vi "CODcr测量数据区.vi"(11 "数组":u16[](array[numeric]) format="%04xH") -> (3 "测量数据区":T1 {"单位" items=["ug/L", "mg/L", "ppm", "mg/m3", "cm", "ppb", "ug/m3", "%", "nmol/mol", "umol/mol", "MPN/L", "MPN/100ml", "ng/m3", "NTU", "无量纲", "ms/cm", "us/cm", "℃", "mV", "万个/L"]})   [LabVIEW 2016, in "CODCr库.lvlib"]
panel:
  # "共占用95 WORD"
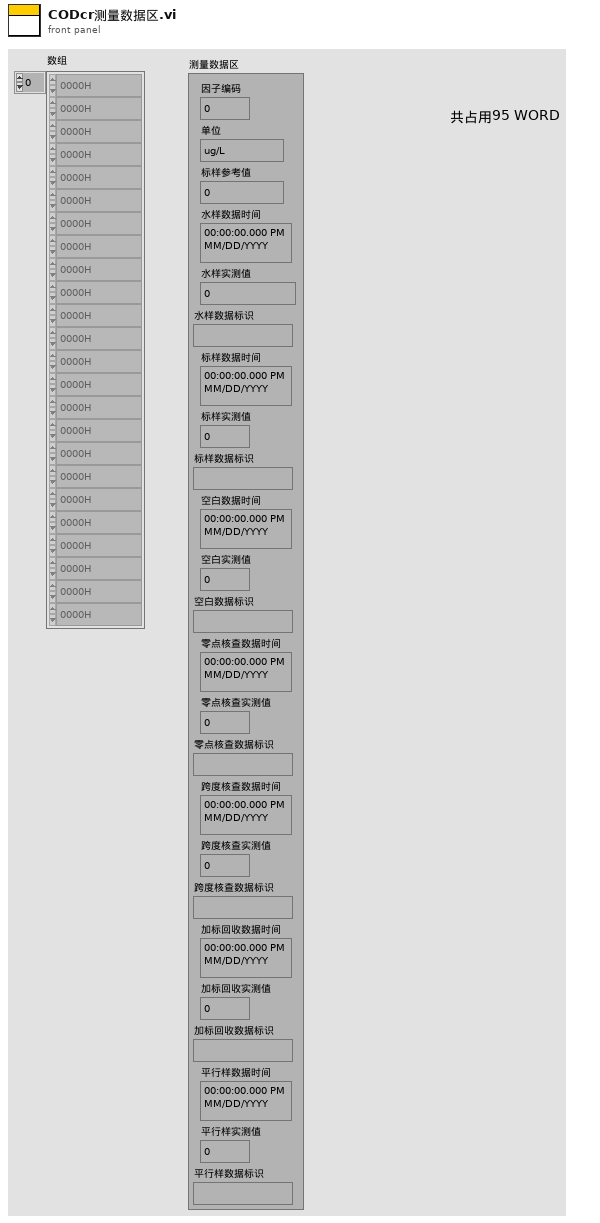
[diagram p1: front panel]
types:
  T1 = cluster{"因子编码":u32, "单位":u16, "标样参考值":sgl, "水样数据时间":timestamp, "水样实测值":sgl, "水样数据标识":string, "标样数据时间":timestamp, "标样实测值":sgl, "标样数据标识":string, "空白数据时间":timestamp, "空白实测值":sgl, "空白数据标识":string, "零点核查数据时间":timestamp, "零点核查实测值":sgl, "零点核查数据标识":string, "跨度核查数据时间":timestamp, "跨度核查实测值":sgl, "跨度核查数据标识":string, "加标回收数据时间":timestamp, "加标回收实测值":sgl, "加标回收数据标识":string, "平行样数据时间":timestamp, "平行样实测值":sgl, "平行样数据标识":string}
  T2 = cluster{"DWORD":i32, "WORD":u16, "FLOAT":sgl, "time stamp":timestamp, "数值":sgl, "string":string, "time stamp":timestamp, "数值":sgl, "string":string, "time stamp":timestamp, "数值":sgl, "string":string, "time stamp":timestamp, "数值":sgl, "string":string, "time stamp":timestamp, "数值":sgl, "string":string, "time stamp":timestamp, "数值":sgl, "string":string, "time stamp":timestamp, "数值":sgl, "string":string}
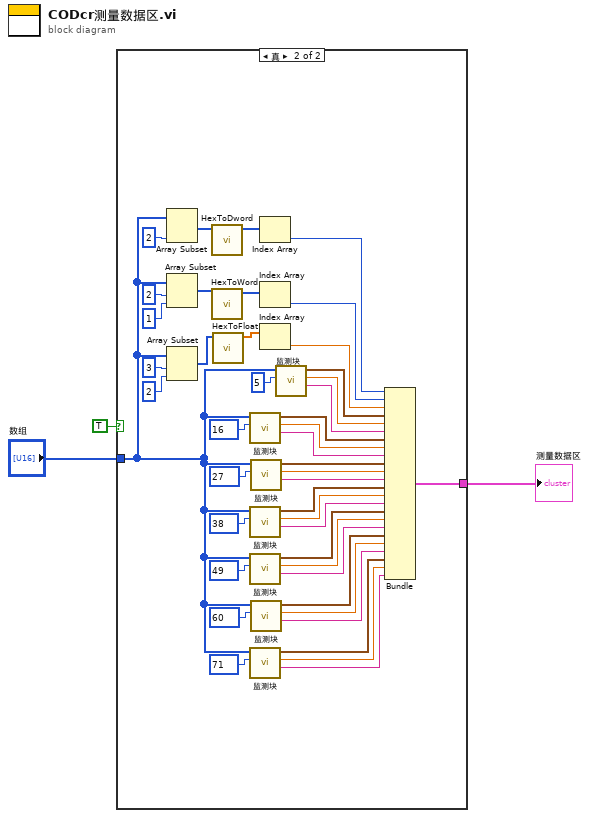
[diagram p0: block diagram]
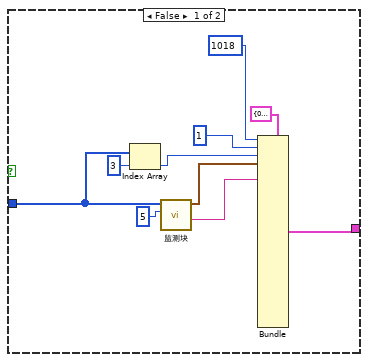
[diagram p2: hidden frame]
diagram:
  n1 = case shown="真" TRUE {
    tunnel: "数组" -> [w7 w22]
    tunnel: [w4 w20] -> w2
    frame False {
      n2 = Index Array(array=w7, index=3 ("索引")) -> (element=w9:u16)
      n3 = call "监测块.vi"("索引"=5, "数组"=w7) -> ("string"=w5:string, "time stamp"=w6:timestamp)  [unwired: 7 in, 1 out]
      n4 = Bundle(cluster=T2 {"DWORD"=0, "WORD"=0, "FLOAT"=0.0, "time stamp"=timestamp(0 s since 1904-01-01), "数值"=0.0, "string"="", "time stamp"=timestamp(0 s since 1904-01-01), "数值"=0.0, "string"="", "time stamp"=timestamp(0 s since 1904-01-01), "数值"=0.0, "string"="", "time stamp"=timestamp(0 s since 1904-01-01), "数值"=0.0, "string"="", "time stamp"=timestamp(0 s since 1904-01-01), "数值"=0.0, "string"="", "time stamp"=timestamp(0 s since 1904-01-01), "数值"=0.0, "string"="", "time stamp"=timestamp(0 s since 1904-01-01), "数值"=0.0, "string"=""}, "DWORD"=1018, "WORD"=u16 1, "FLOAT"=w9, "time stamp"=w6, "string"=w5) -> (w4:T2)  [unwired: 19 in]
    }
    frame True {
      n5 = Array Subset(array=w22, length=2 ("长度")) -> (w19:u16[])  [unwired: 1 in]
      n6 = Array Subset(array=w22, index=2 ("索引"), length=1 ("长度")) -> (w17:u16[])
      n7 = Array Subset(array=w22, index=3 ("索引"), length=2 ("长度")) -> (w15:u16[])
      n8 = call "HexToDword.vi"("数组"=w19) -> ("DWORD"=w18:i32[])  [unwired: 10 in]
      n9 = call "HexToWord.vi"("数组"=w17) -> ("WORD"=w16:u16[])  [unwired: 10 in]
      n10 = call "HexToFloat.vi"("数组"=w15) -> ("FLOAT"=w14:sgl[])  [unwired: 10 in]
      n11 = call "监测块.vi"("索引"=16, "数组"=w22) -> ("string"=w43:string, "数值"=w44:sgl, "time stamp"=w45:timestamp)  [unwired: 7 in]
      n12 = call "监测块.vi"("索引"=38, "数组"=w22) -> ("string"=w35:string, "数值"=w36:sgl, "time stamp"=w37:timestamp)  [unwired: 7 in]
      n13 = call "监测块.vi"("索引"=49, "数组"=w22) -> ("string"=w31:string, "数值"=w32:sgl, "time stamp"=w33:timestamp)  [unwired: 7 in]
      n14 = call "监测块.vi"("索引"=71, "数组"=w22) -> ("string"=w23:string, "数值"=w24:sgl, "time stamp"=w25:timestamp)  [unwired: 7 in]
      n15 = call "监测块.vi"("索引"=27, "数组"=w22) -> ("string"=w39:string, "数值"=w40:sgl, "time stamp"=w41:timestamp)  [unwired: 7 in]
      n16 = call "监测块.vi"("索引"=60, "数组"=w22) -> ("string"=w27:string, "数值"=w28:sgl, "time stamp"=w29:timestamp)  [unwired: 7 in]
      n17 = Index Array(array=w18) -> (element=w21:i32)  [unwired: 1 in]
      n18 = Index Array(array=w16) -> (element=w54:u16)  [unwired: 1 in]
      n19 = Index Array(array=w14) -> (element=w51:sgl)  [unwired: 1 in]
      n20 = call "监测块.vi"("索引"=5, "数组"=w22) -> ("string"=w48:string, "数值"=w49:sgl, "time stamp"=w50:timestamp)  [unwired: 7 in]
      n21 = Bundle("DWORD"=w21, "WORD"=w54, "FLOAT"=w51, "time stamp"=w50, "数值"=w49, "string"=w48, "time stamp"=w45, "数值"=w44, "string"=w43, "time stamp"=w41, "数值"=w40, "string"=w39, "time stamp"=w37, "数值"=w36, "string"=w35, "time stamp"=w33, "数值"=w32, "string"=w31, "time stamp"=w29, "数值"=w28, "string"=w27, "time stamp"=w25, "数值"=w24, "string"=w23) -> (w20:T2)  [unwired: 1 in]
    }
  }
  "测量数据区" <- w2
